vi "数据流读取.vi"() -> ()   [LabVIEW 2016, in "质控单元V2.lvlib"]
panel:
  in  "停止":bool
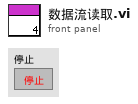
[diagram p1: front panel]
types:
  T1 = typedef "质控单元V2.lvlib/数据流类型.ctl" = cluster{"cmd":enum16{"start", "stop"}, "data":variant}
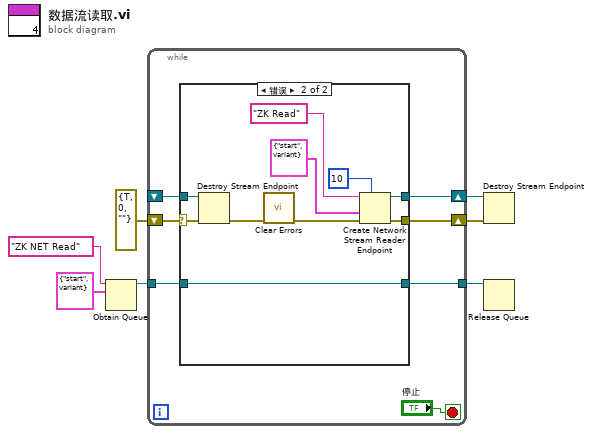
[diagram p0: block diagram]
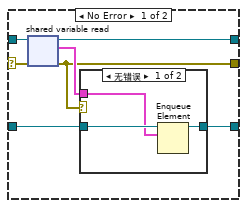
[diagram p2: hidden frame]
diagram:
  n1 = Obtain Queue(name (unnamed)="ZK NET Read" ("名称（未命名）"), element data type=T1 {"cmd"=enum."start", "data"=variant} ("簇")) -> (queue out=w2:refnum<queue>)  [unwired: 3 in, 2 out]
  n2 = while {
    shift-right: [w14] -> w3
    shift-left: errorcluster {"status"=TRUE, "code"=0, "source"=""} ("error out") -> [w13]
    shift-right: [w12] -> w4
    shift-left: _ -> [w11]
    tunnel: w2 -> [w9]
    tunnel: [w8] -> w5
    stop <- "停止" stop-if-true
    n3 = case shown="错误" w13 {
      selector: w13 -> [w20 w32]
      tunnel: [w15 w34] -> w14
      tunnel: [w19 w33] -> w12
      tunnel: w11 -> [w21 w31]
      tunnel: w9 -> [w18 w27]
      tunnel: [w17 w27] -> w8
      frame No Error {
        n4 = shared-variable-read(w21, w20) -> (w19:refnum<k21>, w15:errorcluster, w16:T1)  [unwired: 1 in, 1 out]
        n5 = case shown="无错误" w15 {
          tunnel: w18 -> [w24 w25]
          tunnel: [w23 w25] -> w17
          tunnel: w16 -> [w22 _]
          frame No Error {
            n6 = Enqueue Element(queue=w24, element=w22) -> (queue out=w23:refnum<queue>)  [unwired: 2 in, 2 out]
          }
          frame Error {
          }
        }
      }
      frame Error {
        n7 = Destroy Stream Endpoint(8:w32, 11:w31) -> (0:w30:errorcluster)
        n8 = call <vilib>:"Clear Errors.vi"("error in (no error)"=w30) -> ("error out"=w29:errorcluster)  [unwired: 5 in, 1 out]
        n9 = Create Network Stream Reader Endpoint(7:10 ("写入方缓冲大小"), 8:w29, 9:T1 {"cmd"=enum."start", "data"=variant} ("簇"), 11:"ZK Read" ("写入方名称")) -> (0:w34:errorcluster, 3:w33:refnum<k21>)  [unwired: 3 in]
      }
    }
  }
  n10 = Destroy Stream Endpoint(8:w3, 11:w4) -> ()  [unwired: 1 out]
  n11 = Release Queue(queue=w5) -> ()  [unwired: 2 in, 3 out]
